vi "Database.Cache.NewData.vi"(7 "Idx":i32, 8 "error in":errorcluster, 9 "DBtime":timestamp, 10 "Data":T1 {"Values" format="%.3f"}) -> (0 "error out":errorcluster, 2 "Data saved":bool)   [LabVIEW 2016]
doc: "Write test results (measurement values) to proda database\n\nWabco 2017 All right reserved\nAuthor: maciej.szupienko@wabco-auto.com"
uses:
  Cache/Cache.ProductComponent.Data.ctl
  Tools/EventLog/EventLog.EventSource.ctl
  Tools/Translator/Translator.Message.ctl
  Cache/Cache.Status.Fglb.Action.ctl
  Tools/EventLog/EventLog.New(array).vi
  Drivers/PLC/LowLevel/PLC.DataBlock.PLCvalues.ctl
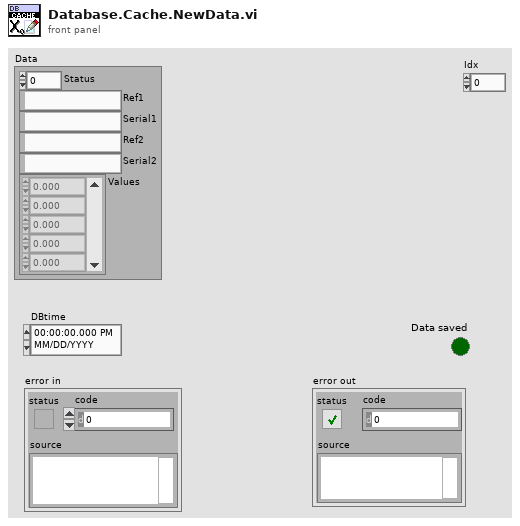
[diagram p1: front panel]
types:
  T1 = typedef "PLC.DataBlock.PLCvalues.ctl" = cluster{"Status":u8, "Ref1":string, "Serial1":string, "Ref2":string, "Serial2":string, "Values":sgl[]}
  T2 = typedef "Cache.Status.Fglb.Action.ctl" = enum16{"init", "Changeover", "CheckStatus", "NewData", "get"}
  T3 = typedef "Translator.Message.ctl" = enum16{"-", "Event confirmed", "Log out", "Log in", "Shutdown", "Cancel", "Start", "Continue", "Stop", "On", "Off", "OK", "NOK", "NOK %s", "This", "Prev", "Home", "Work", "In progress...", "Missing", "Empty", "Hardware failure", "Initial", "Error %d >> %s", "Error %d >> %s >> %s", "Starting %s", "Quitting %s", "Configured", "Initializing", "Quitting", "Loading", "Running %s", "Stopped", "Summary", "Do you want to continue?", "Do you want to exit?", "Log out?", "System", "All", "IDLE", "Translating...%s", "Not found", "Alarm %s", "Run", "Skip", "Abort", "Repeat", "Please wait...", "Database disconnected", "Login to database successful", "Login to database failed: %d; %s", "Get process step data for %s", "Changeover off", "Changeover into %s", "Product %s | %s found in cache with status %d at previous station", "Product %s | %s found in database with status %d at previous station", "Product %s | %s not found in cache at previous station", "Product %s | %s not found in database at previous station", "Product %s | %s found in cache with status %d at this station (%d repetion)", "Product %s | %s found in database with status %d at this station (%d repetition)", "Product %s | %s not found in cache at this station", "Product %s | %s not found in database at this station", "Product %s | %s found in cache for component %s | %s", "Product %s | %s found in database for component %s | %s", "Product not found in cache for component %s | %s", "Product not found in database for component %s | %s", "Product %s | %s connected with component %s | %s (cache)", "Product %s | %s connected with component %s | %s (database)", "New data for %s | %s (cache)", "New data for %s | %s (database)", "File %s moved (cache)", "File %s deleted (cache)", "Msg %d >> %s", "PLC LifeBit Failure", "Reconnecting DB", "Reconnecting PLC", "Free disk space is below 1GB - contact technician", "Unable to check product status", "Product %s SN %s checked in DB", "Unable To check status from station %s"}
  T4 = typedef "EventLog.EventSource.ctl" = enum16{"All", "Gui", "Cache", "PLC1", "PLC2", "PLC3", "DB", "DB01", "DB02", "DB03", "DB04", "DB05", "DB06", "DB07", "DB08", "DB09", "DB10", "DB11", "DB12", "DB13", "DB14", "DB15", "DB16"}
  T5 = typedef "Cache.ProductComponent.Data.ctl" = cluster{"Time":timestamp, "Station":string, "Ref1":string, "Serial1":string, "Ref2":string, "Serial2":string}
  T6 = typedef "Cache.TestSteps.Fglb.ResultData.ctl" = cluster{"File":path, "Ref":string, "Serial":string, "Pr":T7, "PSr":T8, "TSr":cluster{"TSr":T9, "TVr":T10[]}[]}
  T7 = typedef "ProdaNG.ProcessResult.ctl" = cluster{"c_id":string, "productId":string, "processId":i32, "statusId":i32, "startTime":string, "endTime":string}
  T8 = typedef "ProdaNG.ProcessStepResult.ctl" = cluster{"c_id":string, "processResultId":string, "processStepId":i32, "statusId":i32, "operatorId":i32, "startTime":string, "endTime":string}
  T9 = typedef "ProdaNG.TestStepResult.ctl" = cluster{"c_id":string, "processStepResultId":string, "testStepId":i32, "statusId":i32}
  T10 = typedef "ProdaNG.TestValueResult.ctl" = cluster{"c_id":string, "testStepResultId":string, "testValueId":i32, "result":dbl, "statusId":i32, "contentId":string}
  T11 = typedef "Cache.TestSteps.Fglb.TestData.ctl" = cluster{"Ref":string, "Desc":string, "P":T12, "PS":T13, "PP":T14[], "TS":cluster{"TS":T15, "TV":T16[], "TP":T17[]}[], "Units":T18[]}
  T12 = typedef "ProdaNG.Process.ctl" = cluster{"i_id":i32, "productionLineId":i32, "releaseId":i32, "contentId":string, "previewId":string, "mdReason":string, "mdUser":string, "mdTime":string, "description":string}
  T13 = typedef "ProdaNG.ProcessStep.ctl" = cluster{"i_id":i32, "processId":i32, "systemId":i32, "releaseId":i32, "processSequence":i32, "limitYellow":dbl, "limitRed":dbl, "mdReason":string, "mdUser":string, "mdTime":string, "filename":string, "transfer":string, "description":string}
  T14 = typedef "ProdaNG.ProcessStepParam.ctl" = cluster{"i_id":i32, "processStepId":i32, "unitId":i32, "contentId":string, "previewId":string, "value":dbl, "valueText":string, "paramSequence":i32, "history":i32, "mdReason":string, "mdUser":string, "mdTime":string, "description":string}
  T15 = typedef "ProdaNG.TestStep.ctl" = cluster{"i_id":i32, "processStepId":i32, "testSequence":i32, "testOrder":i32, "mdReason":string, "mdUser":string, "mdTime":string, "description":string}
  T16 = typedef "ProdaNG.TestValue.ctl" = cluster{"i_id":i32, "testStepId":i32, "releaseId":i32, "unitId":i32, "contentId":string, "previewId":string, "maximum":dbl, "minimum":dbl, "valueText":string, "testValueSequence":i32, "history":i32, "mdReason":string, "mdUser":string, "mdTime":string, "description":string}
  T17 = typedef "ProdaNG.TestStepParam.ctl" = cluster{"i_id":i32, "testStepId":i32, "unitId":i32, "contentId":string, "previewId":string, "value":dbl, "valueText":string, "paramSequence":i32, "history":i32, "mdReason":string, "mdUser":string, "mdTime":string, "description":string}
  T18 = typedef "ProdaNG.Unit.ctl" = cluster{"i_id":i32, "name":string, "mdReason":string, "mdUser":string, "mdTime":string, "description":string}
  T19 = typedef "Database.Data.Sets.ctl" = cluster{"Enable":bool, "ConnString":string, "SystemName":string, "Process.Begin":bool, "Process.End":bool}
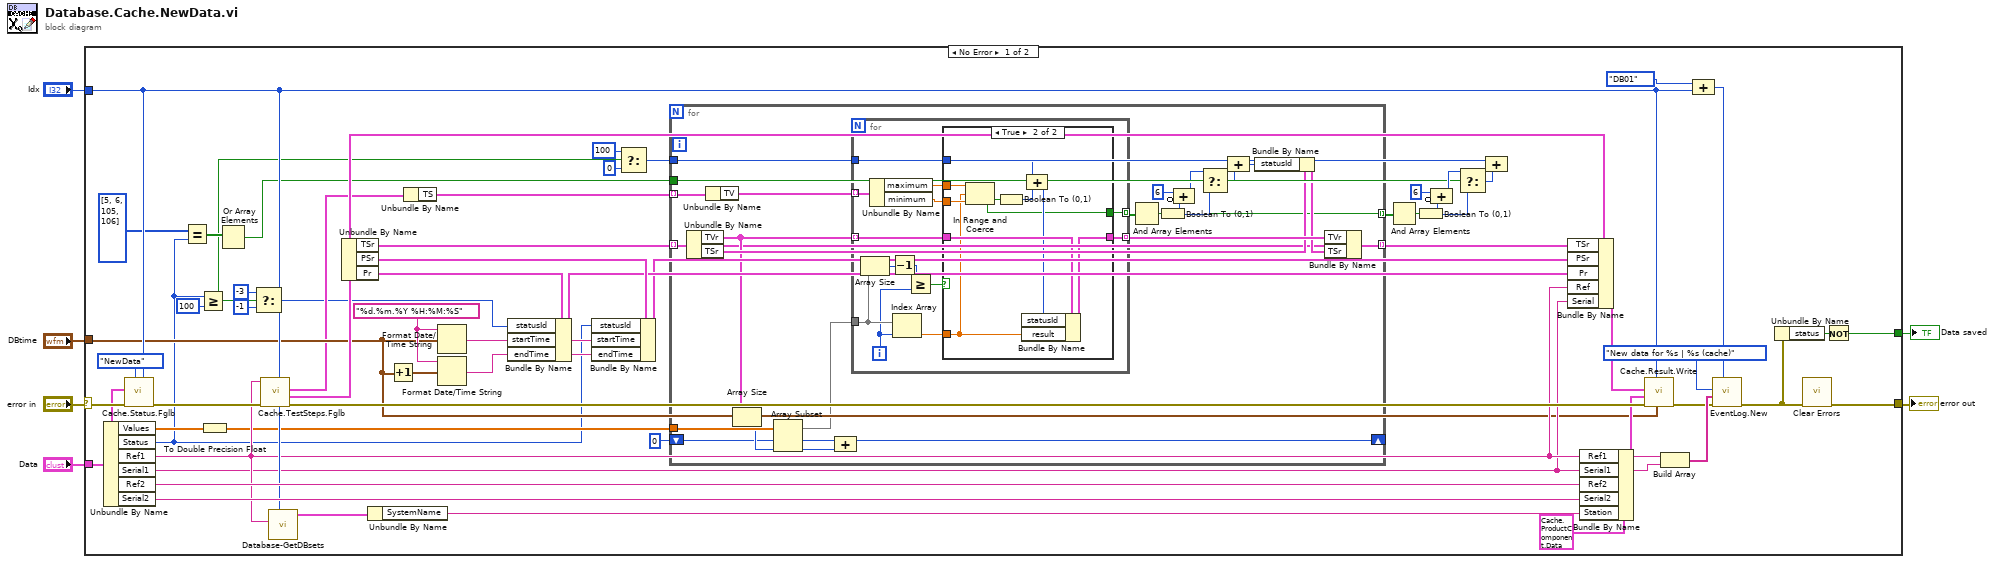
[diagram p0: block diagram]
diagram:
  n1 = case shown="No Error" "error in" {
    selector: "error in" -> [w40 w111]
    tunnel: [w54 w111] -> w6
    tunnel: "Data" -> [w37 _]
    tunnel: "Idx" -> [w34 _]
    tunnel: [w52 _] -> w3
    tunnel: "DBtime" -> [w29 _]
    frame No Error {
      w61 = "%d.%m.%Y %H:%M:%S" ("time format string (%c)")
      n2 = Unbundle By Name(w37) -> ("Values"=w65:sgl[], "Status"=w7:u8, "Ref1"=w33:string, "Serial1"=w32:string, "Ref2"=w49:string, "Serial2"=w50:string)
      n3 = call "Cache.Status.Fglb.vi"("SystemIdx"=w34, "Action (get)"=Cache.Status.Fglb.Action."NewData", "error in (no error)"=w40, "NewData"=w37) -> ("error out"=w39:errorcluster)  [unwired: 6 in, 1 out]
      n4 = Equal?(x=u8[] [5, 6, 105, 106], y=w7) -> (x = y?=w23:bool[])
      n5 = Greater Or Equal?(x=w7, y=u8 100) -> (x >= y?=w14:bool)
      n6 = To Double Precision Float(number=w65) -> (double precision float=w25:dbl[])
      n7 = Or Array Elements(Boolean array=w23) -> (logical OR=w10:bool)
      n8 = Select(t=-3 ("statusId"), s=w14, f=-1 ("statusId")) -> (s? t:f=w12:i32)
      n9 = call "Cache.TestSteps.Fglb.vi"("SystemIdx"=w34, "error in (no error)"=w39, "Variant"=w33) -> ("error out"=w55:errorcluster, "Result out"=w57:T6, "Test out"=w27:T11)  [unwired: 5 in, 1 out]
      n10 = call "Database-GetDBsets.vi"("Idx"=w34, "Variant"=w33) -> ("Sets"=w35:T19)  [unwired: 5 in, 4 out]
      n11 = Unbundle By Name(w57) -> ("TSr"=w64:cluster{"TSr":T9, "TVr":T10[]}[], "PSr"=w63:T8, "Pr"=w11:T7)
      n12 = Unbundle By Name(w35) -> ("SystemName"=w28:string)
      n13 = Increment(x=w29) -> (x+1=w60:timestamp)
      n14 = Unbundle By Name(w27) -> ("TS"=w26:cluster{"TS":T15, "TV":T16[], "TP":T17[]}[])
      n15 = Format Date/Time String(time format string (%c)=w61, seconds (now)=w29) -> (date/time string=w59:string)  [unwired: 1 in]
      n16 = Format Date/Time String(time format string (%c)=w61, seconds (now)=w60) -> (date/time string=w58:string)  [unwired: 1 in]
      n17 = Bundle By Name(cluster=w11, "statusId"=w12, "startTime"=w59, "endTime"=w58) -> (w9:T7)
      n18 = Bundle By Name(cluster=w63, "statusId"=w7, "startTime"=w59, "endTime"=w58) -> (w8:T8)
      n19 = Select(t=100 ("0, 1"), s=w14, f=0 ("0, 1")) -> (s? t:f=w13:i32)
      n20 = for {
        tunnel: w25 -> [w84]
        tunnel: w64 -> [w66] mode=indexing
        tunnel: [w85] -> w56 mode=indexing
        shift-right: [w79] -> _
        shift-left: 0 -> [w81]
        tunnel: w26 -> [w76] mode=indexing
        tunnel: w13 -> [w67]
        tunnel: w10 -> [w74]
        tunnel: [w68] -> w17 mode=indexing
        n21 = Unbundle By Name(w66) -> ("TVr"=w83:T10[], "TSr"=w86:T9)
        n22 = Unbundle By Name(w76) -> ("TV"=w77:T16[])
        n23 = Array Size(array=w83) -> (size(s)=w82:i32)
        n24 = Array Subset(array=w84, index=w81, length=w82) -> (w80:dbl[])
        n25 = Compound Arithmetic op=ADD(w81, w82) -> (w79:i32)
        n26 = for "results" {
          tunnel: w80 -> [w95]
          tunnel: w83 -> [w100] mode=indexing
          tunnel: [w99] -> w87 mode=indexing
          tunnel: w77 -> [w93] mode=indexing
          tunnel: w67 -> [w89]
          tunnel: [w88] -> w75 mode=indexing
          i -> [w94]
          n27 = Array Size(array=w95) -> (size(s)=w96:i32)
          n28 = Unbundle By Name(w93) -> ("maximum"=w92:dbl, "minimum"=w91:dbl)
          n29 = Decrement(x=w96) -> (x-1=w90:i32)
          n30 = Index Array(array=w95, index=w94) -> (element=w98:dbl)
          n31 = Greater Or Equal?(x=w90, y=w94) -> (x >= y?=w97:bool)
          n32 = case shown="True" w97 {
            tunnel: w100 -> [w101 w110]
            tunnel: [w101 w109] -> w99
            tunnel: w98 -> [_ w106]
            tunnel: w92 -> [_ w108]
            tunnel: w91 -> [_ w107]
            tunnel: w89 -> [_ w102]
            tunnel: [_ w103] -> w88
            frame False {
            }
            frame True {
              n33 = In Range and Coerce(upper limit=w108, x=w106, lower limit=w107) -> (In Range?=w103:bool)  [unwired: 1 out]
              n34 = Boolean To (0,1)(Boolean=w103) -> (0, 1=w105:i16)
              n35 = Compound Arithmetic op=ADD(w102, w105) -> (w104:i32)
              n36 = Bundle By Name(cluster=w110, "statusId"=w104, "result"=w106) -> (w109:T10)
            }
          }
        }
        n37 = And Array Elements(Boolean array=w75) -> (logical AND=w68:bool)
        n38 = Boolean To (0,1)(Boolean=w68) -> (0, 1=w73:i16)
        n39 = Compound Arithmetic op=ADD(i16 6 ("0, 1"), invert w73) -> (w71:i16)
        n40 = Select(t=w71, s=w74, f=w73) -> (s? t:f=w70:i16)
        n41 = Compound Arithmetic op=unknown(w67, w70) -> (w69:i32)
        n42 = Bundle By Name(cluster=w86, "statusId"=w69) -> (w78:T9)
        n43 = Bundle By Name(cluster=w66, "TVr"=w87, "TSr"=w78) -> (w85:cluster{"TSr":T9, "TVr":T10[]})
      }
      n44 = And Array Elements(Boolean array=w17) -> (logical AND=w18:bool)
      n45 = Boolean To (0,1)(Boolean=w18) -> (0, 1=w19:i16)
      n46 = Compound Arithmetic op=ADD(i16 6 ("0, 1"), invert w19) -> (w21:i16)
      n47 = Select(t=w21, s=w10, f=w19) -> (s? t:f=w22:i16)
      n48 = Compound Arithmetic op=ADD(w13, w22) -> ()  [unwired: 1 out]
      n49 = Bundle By Name(cluster=w57, "TSr"=w56, "PSr"=w8, "Pr"=w9, "Ref"=w33, "Serial"=w32) -> (w36:T6)
      n50 = Bundle By Name(cluster=T5 {"Time"=timestamp(0 s since 1904-01-01), "Station"="", "Ref1"="", "Serial1"="", "Ref2"="", "Serial2"=""} ("ProdComp"), "Ref1"=w33, "Serial1"=w32, "Ref2"=w49, "Serial2"=w50, "Station"=w28) -> (w30:T5)
      n51 = call "Cache.Result.Write.vi"("Time (now)"=w29, "Idx"=w34, "error in (no error)"=w55, "ProdComp"=w30, "Result in"=w36) -> ("error out"=w31:errorcluster)  [unwired: 5 in, 1 out]
      n52 = Build Array(w33, w32) -> (w41:string[])
      n53 = Compound Arithmetic op=ADD(EventLog.EventSource."DB01" ("Source (All)"), w34) -> (w44:i32)
      n54 = call-poly "EventLog.New.vi"("Source (All)"=w44, "error in (no error)"=w31, "Arguments"=w41, "Message (-)"=Translator.Message."New data for %s | %s (cache)") -> ("error out"=w43:errorcluster)  [unwired: 6 in, 1 out]
      n55 = Unbundle By Name(w43) -> ("status"=w53:bool)
      n56 = call <vilib>:"Clear Errors.vi"("error in (no error)"=w43) -> ("error out"=w54:errorcluster)  [unwired: 5 in, 1 out]
      n57 = Not(x=w53) -> (.not. x?=w52:bool)
    }
    frame Error {
    }
  }
  "error out" <- w6
  "Data saved" <- w3
